vi "Transition EMS.vi"(8 "error in":errorcluster, 11 "Master Controller in":refnum<class "EMS User Interface.lvclass">) -> (0 "error out":errorcluster, 3 "Master Controller out":refnum<class "EMS User Interface.lvclass">)   [LabVIEW 2018, in "EMS User Interface Actor.lvlib" / "EMS User Interface.lvclass"]
uses:
  EMS User Interface.lvclass
  EMS User Interface.lvclass/EMS User Interface.ctl
  <vilib>/ActorFramework/Message Enqueuer/Message Enqueuer.lvclass/Message Enqueuer.ctl
  <vilib>/ActorFramework/Message Enqueuer/Enqueue.vi
  EMS Core/EMS Messages/Resynchronization Init Msg/Resynchronization Init Msg.lvclass
  C:/Program Files (x86)/National Instruments/LabVIEW 2018/vi.lib/ActorFramework/Message/Message.lvclass
  EMS Core/EMS Messages/Island Init Msg/Island Init Msg.lvclass
  <vilib>/ActorFramework/Message Priority Queue/Priority Enqueue.vi
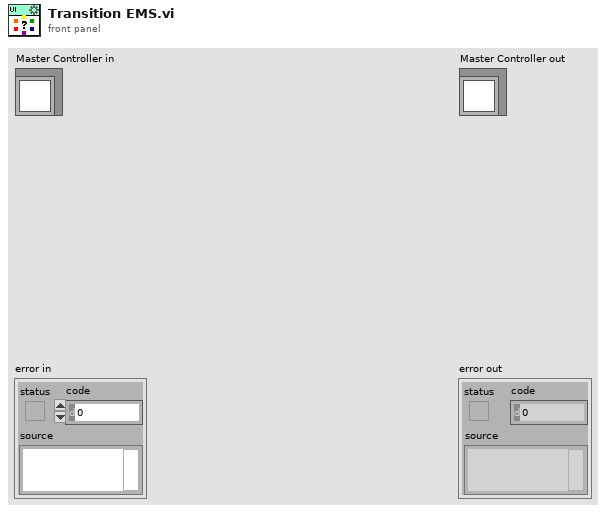
[diagram p1: front panel]
types:
  T1 = typedef "EMS Core.lvlib/EMS.lvclass/Microgrid State.ctl" = enum16{"Discovery", "Commissioning", "Activation", "Blackstart", "OnGrid", "OffGrid", "Island", "Resynchronization", "Manual", "Shutdown", "Stop"}
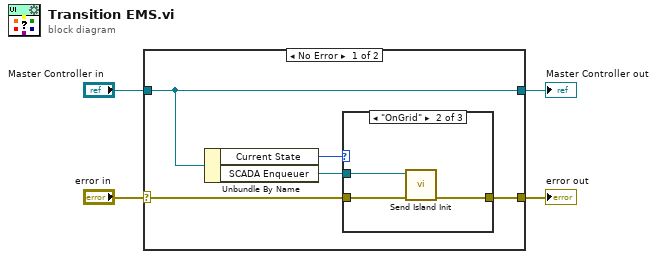
[diagram p0: block diagram]
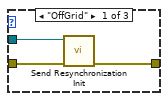
[diagram p2: hidden frame]
diagram:
  n1 = case shown="No Error" "error in" {
    selector: "error in" -> [w6 w18]
    tunnel: [w5 w18] -> w3
    tunnel: [w9 w17] -> w1
    tunnel: "Master Controller in" -> [w9 w17]
    frame No Error {
      n2 = Unbundle By Name(w9) -> ("Current State"=w8:T1, "SCADA Enqueuer"=w7:refnum<class "Message Enqueuer.lvclass">)
      n3 = case shown="\"OnGrid\"" w8 {
        tunnel: w7 -> [w11 w15 _]
        tunnel: w6 -> [w12 w14 w16]
        tunnel: [w10 w13 w16] -> w5
        frame "OffGrid" {
          n4 = call "Send Resynchronization Init.vi"("error in (no error)"=w12, "Message Enqueuer"=w11) -> ("error out"=w10:errorcluster)  [unwired: 8 in, 1 out]
        }
        frame "OnGrid" {
          n5 = call "Send Island Init.vi"("error in (no error)"=w14, "Message Enqueuer"=w15) -> ("error out"=w13:errorcluster)  [unwired: 8 in, 1 out]
        }
        frame "Commissioning", Default {
        }
      }
    }
    frame Error {
    }
  }
  "error out" <- w3
  "Master Controller out" <- w1
